vi "ServoMotor.vi"() -> ()   [LabVIEW 2023]
uses:
  <vilib>/Instr/_visa.llb/VISA Configure Serial Port (Instr).vi
panel:
  in  "stop":bool
  in  "VISA resource name":refnum<visa-resource-name>
  in  "GRADOS":dbl(knob) scale=0.0..180.0
  # "SERVOMOTOR"
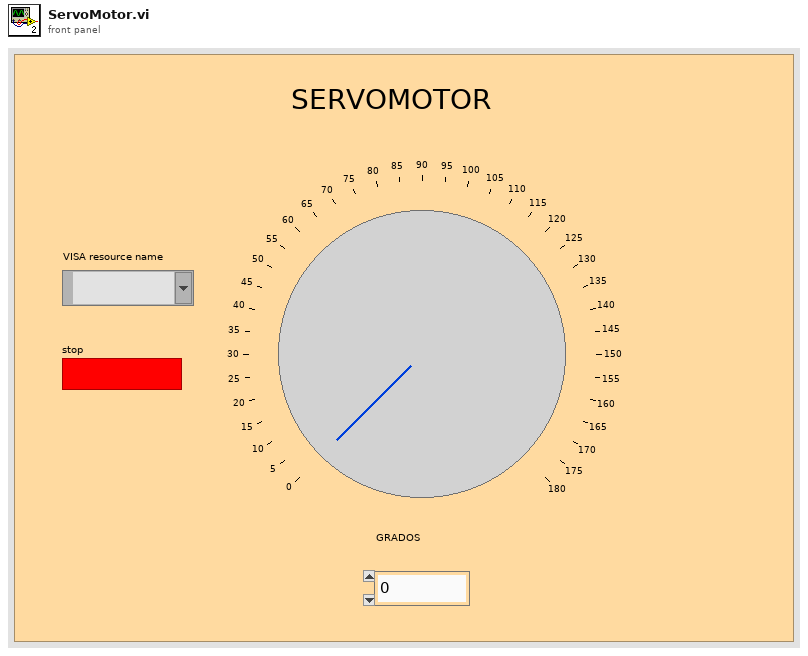
[diagram p1: front panel]
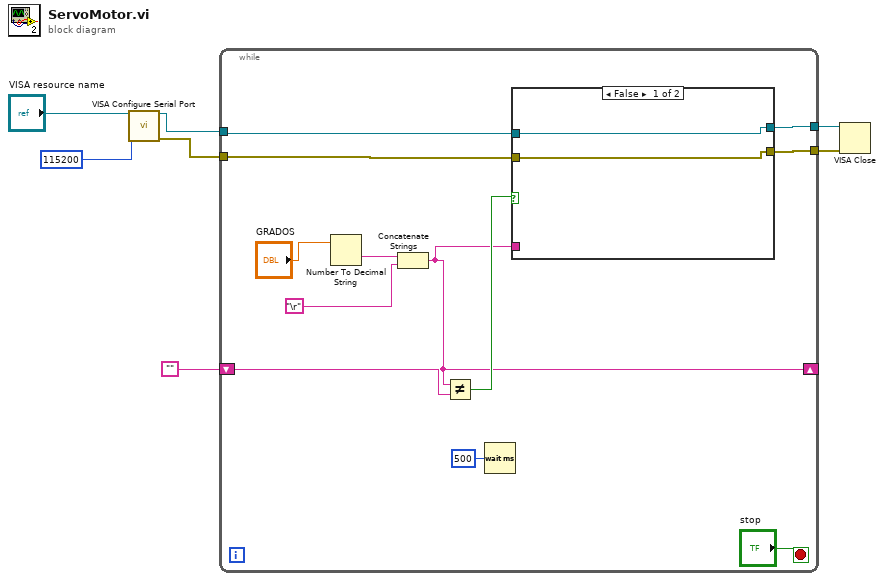
[diagram p0: block diagram]
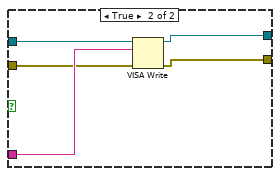
[diagram p2: hidden frame]
diagram:
  n1 = call-poly "VISA Configure Serial Port"("VISA resource name"="VISA resource name", "baud rate (9600)"=u32 115200) -> ("VISA resource name out"=w5:refnum<visa-resource-name>, "error out"=w1:errorcluster)  [unwired: 12 in]
  n2 = while {
    tunnel: w5 -> [w14]
    tunnel: [w19] -> w4
    tunnel: [w18] -> w3
    shift-right: [w10] -> _
    shift-left: "" -> [w11]
    tunnel: w1 -> [w13]
    stop <- "stop" stop-if-true
    n3 = Number To Decimal String(number="GRADOS") -> (decimal integer string=w16:string)  [unwired: 1 in]
    n4 = Concatenate Strings(w16, "\r") -> (w10:string)
    n5 = Not Equal?(x=w10, y=w11) -> (x != y?=w12:bool)
    n6 = Wait (ms)(milliseconds to wait=u32 500) -> ()  [unwired: 1 out]
    n7 = case shown="False" w12 {
      tunnel: [w21 w26] -> w19
      tunnel: [w20 w25] -> w18
      tunnel: w10 -> [_ w24]
      tunnel: w14 -> [w21 w23]
      tunnel: w13 -> [w20 w22]
      frame False {
      }
      frame True {
        n8 = VISA Write(VISA resource name=w23, write buffer=w24, error in (no error)=w22) -> (VISA resource name out=w26:refnum<visa-resource-name>, error out=w25:errorcluster)  [unwired: 1 out]
      }
    }
  }
  n9 = VISA Close(VISA resource name=w4, error in (no error)=w3) -> ()  [unwired: 1 out]
